vi "Delete Element From Array of TA Binding.vi"(10 "index":i32, 11 "Motions in":refnum<class "Motions.lvclass">) -> (3 "Motions out":refnum<class "Motions.lvclass">)   [LabVIEW 2016, in "Hardware.lvlib" / "Motions.lvlib" / "Motions.lvclass"]
uses:
  <userlib>/Common Components/Hardware/Abstract System/Motions/Motions/Motions.lvclass
  <userlib>/Common Components/Hardware/Abstract System/Motions/Motions/Motions.lvclass/Motions.ctl
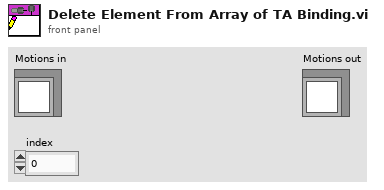
[diagram p1: front panel]
types:
  T1 = typedef "Hardware.lvlib/Motions.lvlib/Motions.lvclass/TA Binding Data.ctl" = cluster{"Triggers":cluster{"Triggers for Array AND":cluster{"Index":u8, "State Name":string}[]}[], "Actions":cluster{"Action Name":string, "Action Data":string}[]}
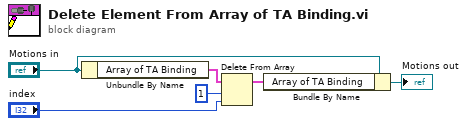
[diagram p0: block diagram]
diagram:
  n1 = Unbundle By Name("Motions in") -> ("Array of TA Binding"=w4:T1[])
  n2 = Delete From Array(array=w4, length=1, index="index") -> (array with subset deleted=w3:T1[])  [unwired: 1 out]
  n3 = Bundle By Name(cluster="Motions in", "Array of TA Binding"=w3) -> (→"Motions out":refnum<class "Motions.lvclass">)
